vi "Set Registers.vi"(0 "VISA Resource Name":refnum<visa-resource-name>, 5 "Reg (15:dq STATUS GROUP: EVENT)":T1(ring)=enum."dq STATUS GROUP: EVENT", 9 "Register Data (0)":u16, 11 "error in (no error)":errorcluster {"code" format="%.0x"}) -> (4 "VISA Resource Name Out":refnum<visa-resource-name>, 15 "error out":errorcluster {"code" format="%.0x"})   [LabVIEW 2012, in "Agilent ESG Series.lvlib"]
doc: "This VI is used set the data within a specified register."
uses:
  <instrlib>/Agilent ESG Series/Agilent ESG Series.lvlib
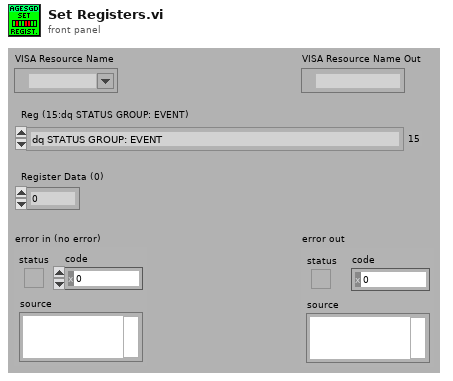
[diagram p1: front panel]
types:
  T1 = enum16{"dq BERT STATUS GROUP: EVENT", "dq BERT STATUS GROUP: NEGATIVE TRANSITION FILTER", "dq BERT STATUS GROUP: POSITIVE TRANSITION FILTER", "dq CALIBRATION STATUS GROUP: EVENT", "dq CALIBRATION STATUS GROUP: NEGATIVE TRANSITION FILTER", "dq CALIBRATION STATUS GROUP: POSITIVE TRANSITION FILTER", "dq FREQUENCY STATUS GROUP: EVENT", "dq FREQUENCY STATUS GROUP: NEGATIVE TRANSITION FILTER", "dq FREQUENCY STATUS GROUP: POSITIVE TRANSITION FILTER", "dq MODULATION STATUS GROUP: EVENT", "dq MODULATION STATUS GROUP: NEGATIVE TRANSITION FILTER", "dq MODULATION STATUS GROUP: POSITIVE TRANSITION FILTER", "dq POWER STATUS GROUP: EVENT", "dq POWER STATUS GROUP: NEGATIVE TRANSITION FILTER", "dq POWER STATUS GROUP: POSITIVE TRANSITION FILTER", "dq STATUS GROUP: EVENT", "dq STATUS GROUP: NEGATIVE TRANSITION FILTER", "dq STATUS GROUP: POSITIVE TRANSITION FILTER", "so STATUS GROUP: EVENT", "so STATUS GROUP: NEGATIVE TRANSITION FILTER", "so STATUS GROUP: POSITIVE TRANSITION FILTER"}
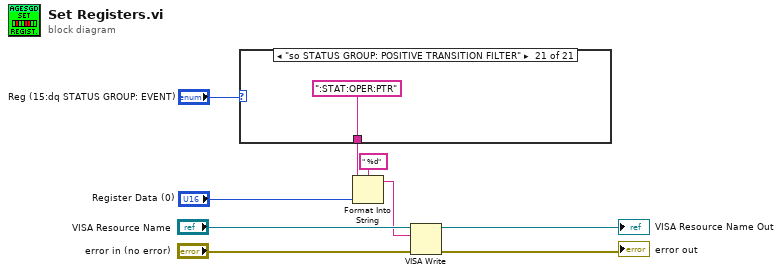
[diagram p0: block diagram]
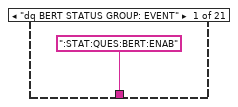
[diagram p2: hidden frame]
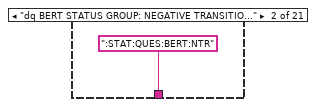
[diagram p3: hidden frame]
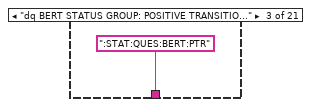
[diagram p4: hidden frame]
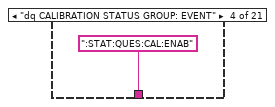
[diagram p5: hidden frame]
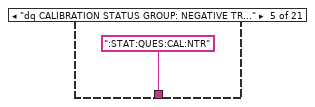
[diagram p6: hidden frame]
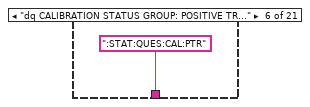
[diagram p7: hidden frame]
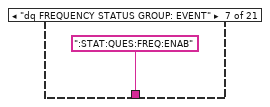
[diagram p8: hidden frame]
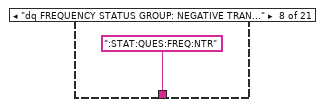
[diagram p9: hidden frame]
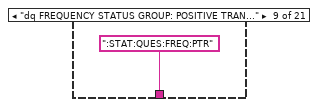
[diagram p10: hidden frame]
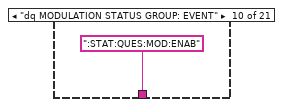
[diagram p11: hidden frame]
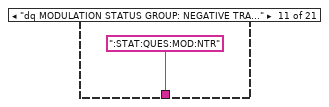
[diagram p12: hidden frame]
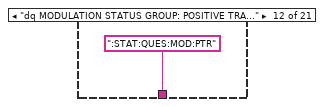
[diagram p13: hidden frame]
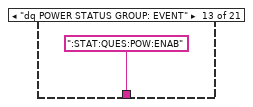
[diagram p14: hidden frame]
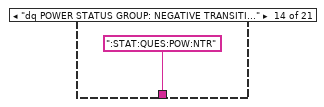
[diagram p15: hidden frame]
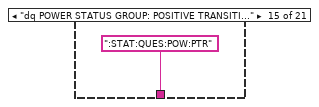
[diagram p16: hidden frame]
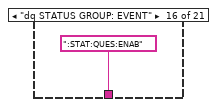
[diagram p17: hidden frame]
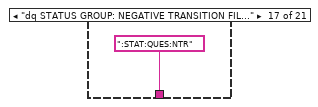
[diagram p18: hidden frame]
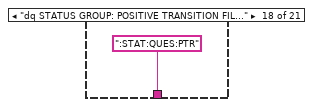
[diagram p19: hidden frame]
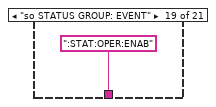
[diagram p20: hidden frame]
diagram:
  n1 = case shown="\"so STATUS GROUP: POSITIVE TRANSITION FILTER\"" "Reg (15:dq STATUS GROUP: EVENT)" {
    tunnel: [":STAT:QUES:BERT:ENAB" ":STAT:QUES:BERT:NTR" ":STAT:QUES:BERT:PTR" ":STAT:QUES:CAL:ENAB" ":STAT:QUES:CAL:NTR" ":STAT:QUES:CAL:PTR" ":STAT:QUES:FREQ:ENAB" ":STAT:QUES:FREQ:NTR" ":STAT:QUES:FREQ:PTR" ":STAT:QUES:MOD:ENAB" ":STAT:QUES:MOD:NTR" ":STAT:QUES:MOD:PTR" ":STAT:QUES:POW:ENAB" ":STAT:QUES:POW:NTR" ":STAT:QUES:POW:PTR" ":STAT:QUES:ENAB" ":STAT:QUES:NTR" ":STAT:QUES:PTR" ":STAT:OPER:ENAB" ":STAT:OPER:NTR" ":STAT:OPER:PTR"] -> w5
    frame "dq BERT STATUS GROUP: EVENT" {
    }
    frame "dq BERT STATUS GROUP: NEGATIVE TRANSITION FILTER" {
    }
    frame "dq BERT STATUS GROUP: POSITIVE TRANSITION FILTER" {
    }
    frame "dq CALIBRATION STATUS GROUP: EVENT" {
    }
    frame "dq CALIBRATION STATUS GROUP: NEGATIVE TRANSITION FILTER" {
    }
    frame "dq CALIBRATION STATUS GROUP: POSITIVE TRANSITION FILTER" {
    }
    frame "dq FREQUENCY STATUS GROUP: EVENT" {
    }
    frame "dq FREQUENCY STATUS GROUP: NEGATIVE TRANSITION FILTER" {
    }
    frame "dq FREQUENCY STATUS GROUP: POSITIVE TRANSITION FILTER" {
    }
    frame "dq MODULATION STATUS GROUP: EVENT" {
    }
    frame "dq MODULATION STATUS GROUP: NEGATIVE TRANSITION FILTER" {
    }
    frame "dq MODULATION STATUS GROUP: POSITIVE TRANSITION FILTER" {
    }
    frame "dq POWER STATUS GROUP: EVENT" {
    }
    frame "dq POWER STATUS GROUP: NEGATIVE TRANSITION FILTER" {
    }
    frame "dq POWER STATUS GROUP: POSITIVE TRANSITION FILTER" {
    }
    frame "dq STATUS GROUP: EVENT" {
    }
    frame "dq STATUS GROUP: NEGATIVE TRANSITION FILTER" {
    }
    frame "dq STATUS GROUP: POSITIVE TRANSITION FILTER" {
    }
    frame "so STATUS GROUP: EVENT" {
    }
    frame "so STATUS GROUP: NEGATIVE TRANSITION FILTER" {
    }
    frame "so STATUS GROUP: POSITIVE TRANSITION FILTER" {
    }
  }
  n2 = Format Into String(format string=" %d", initial string=w5, "Register Data (0)") -> (resulting string=w4:string)  [unwired: 1 in, 1 out]
  n3 = VISA Write(VISA resource name="VISA Resource Name", write buffer=w4, error in (no error)="error in (no error)") -> (VISA resource name out=→"VISA Resource Name Out":refnum<visa-resource-name>, error out=→"error out":errorcluster)  [unwired: 1 out]
